vi "Service_Call_Entry.vi"() -> ()   [LabVIEW 2023]
panel:
  out "Previous Call No.":string
  in  "Submit":bool
  in  "Item Description":string
  in  "Return":bool
  in  "Customer Contact No.":string
  in  "Engineer Name":string
  in  "Problem":string
  in  "Customer":string
  in  "Call No.":string
  # "SERvice call entry"
  # "UTKARSH ENTERPRISES"
  # "Developed By- Samarth Wagh (waghsamarth@gmail.com) 7972965098"
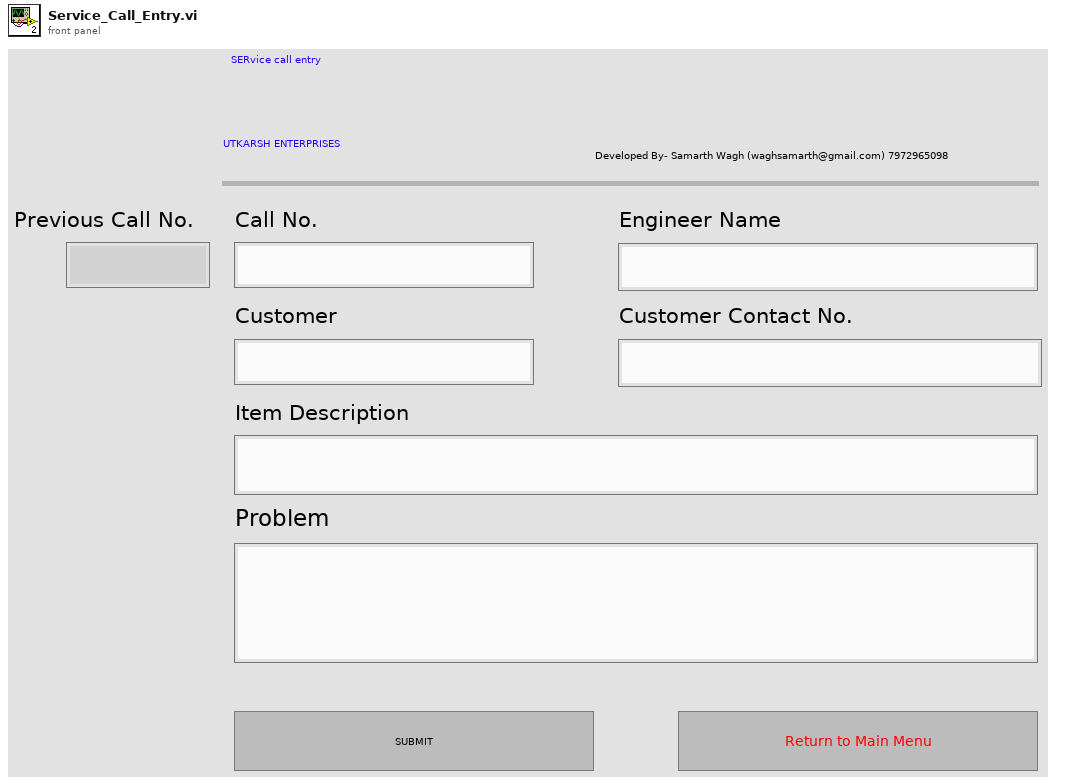
[diagram p1: front panel]
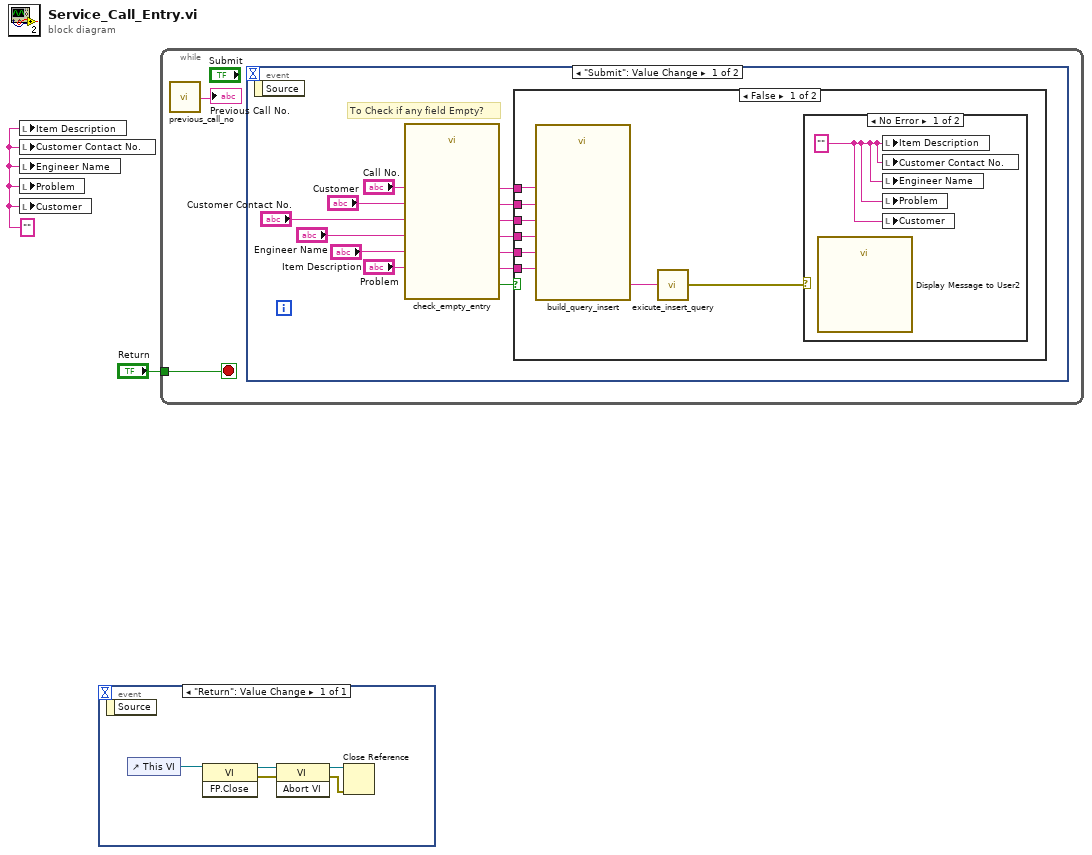
[diagram p0: block diagram]
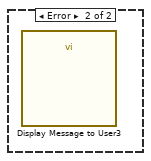
[diagram p2: hidden frame]
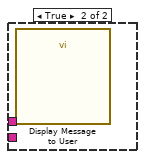
[diagram p3: hidden frame]
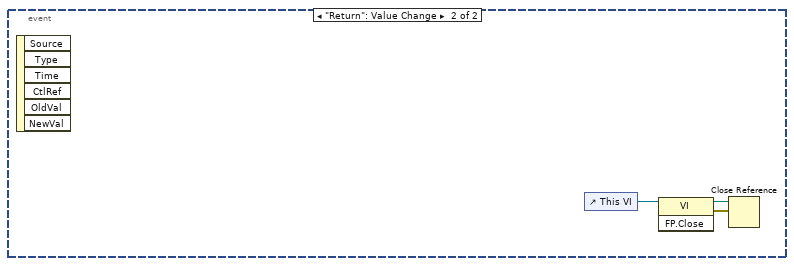
[diagram p4: hidden frame]
diagram:
  w2 = ""
  n1 = local write "Item Description"(w2) -> ()
  n2 = local write "Customer Contact No."(w2) -> ()
  n3 = local write "Engineer Name"(w2) -> ()
  n4 = local write "Problem"(w2) -> ()
  n5 = local write "Customer"(w2) -> ()
  n6 = event shown="[0] \"Return\": Value Change" {
    selector: _ -> [_]
    dyn-events: _ -> [_]
    timeout: _ -> [_]
    event "Return": Value Change {
      n7 = event-data() -> ()  [unwired: 1 in, 1 out]
      n8 = control-ref of="This VI"() -> (w7:refnum<vi>)
      n9 = invoke class="VI" method="FP.Close"(reference=w7) -> (reference out=w6:refnum<vi>, error out=w5:errorcluster)  [unwired: 2 in, 1 out]
      n10 = invoke class="VI" method="Abort VI"(reference=w6, error in=w5) -> (reference out=w3:refnum<vi>, error out=w4:errorcluster)  [unwired: 1 in, 1 out]
      n11 = Close Reference(reference=w3, error in (no error)=w4) -> ()  [unwired: 1 out]
    }
  }
  n12 = while {
    tunnel: "Return" -> [w9]
    stop <- w9 stop-if-true
    n13 = call "previous_call_no.vi"() -> ("Previous Call No."=→"Previous Call No.":string)  [unwired: 11 in]
    n14 = event shown="[0] \"Submit\": Value Change" {
      selector: _ -> [_ _]
      dyn-events: _ -> [_ _]
      timeout: _ -> [_ _]
      event "Submit": Value Change {
        # "To Check if any field Empty?"
        n15 = event-data() -> ()  [unwired: 1 in, 1 out]
        n16 = call "check_empty_entry.vi"("Problem"="Problem", "Customer Contact No."="Customer Contact No.", "Call No."="Call No.", "Engineer Name"="Engineer Name", "Item Description"="Item Description", "Customer"="Customer") -> ("Boolean"=w16:bool)  [unwired: 5 in]
        n17 = case shown="False" w16 {
          tunnel: "Call No." -> [w24 _]
          tunnel: "Engineer Name" -> [w23 _]
          tunnel: "Problem" -> [w19 _]
          tunnel: "Customer" -> [w22 _]
          tunnel: "Item Description" -> [w20 _]
          tunnel: "Customer Contact No." -> [w21 _]
          frame False {
            n18 = call "build_query_insert.vi"("Problem"=w19, "Item Description"=w20, "Call No."=w24, "Customer Contact No."=w21, "Customer"=w22, "Engineer Name"=w23) -> ("result string"=w18:string)  [unwired: 5 in]
            n19 = call "exicute_insert_query.vi"("result string"=w18) -> ("error out"=w17:errorcluster)  [unwired: 10 in]
            n20 = case shown="No Error" w17 {
              frame No Error {
                w25 = ""
                n21 = call "Display Message to User2"() -> ()  [unwired: 10 in, 2 out]
                n22 = local write "Item Description"(w25) -> ()
                n23 = local write "Customer Contact No."(w25) -> ()
                n24 = local write "Engineer Name"(w25) -> ()
                n25 = local write "Problem"(w25) -> ()
                n26 = local write "Customer"(w25) -> ()
              }
              frame Error {
                n27 = call "Display Message to User3"() -> ()  [unwired: 10 in, 2 out]
              }
            }
          }
          frame True {
            n28 = call "Display Message to User"() -> ()  [unwired: 10 in, 2 out]
          }
        }
      }
      event "Return": Value Change {
        n29 = event-data() -> ()  [unwired: 1 in, 6 out]
        n30 = control-ref of="This VI"() -> (w26:refnum<vi>)
        n31 = invoke class="VI" method="FP.Close"(reference=w26) -> (reference out=w27:refnum<vi>, error out=w28:errorcluster)  [unwired: 2 in, 1 out]
        n32 = Close Reference(reference=w27, error in (no error)=w28) -> ()  [unwired: 1 out]
      }
    }
  }
